vi "VIQA Find Legal Marking.vi"(8 "error in (no error)":errorcluster, 9 "Return Decor Refnum? (F)":bool, 10 "Ignore? (F)":bool, 11 "VI Refnum":refnum<vi>) -> (0 "error out":errorcluster, 1 "Found?":bool, 2 "Legal Marking":string, 3 "dup VI Refnum":refnum<vi>, 5 "Decor Refnum":refnum<vi>, 7 "Tag Name":string="BATC_SW_LEGALMARKING")   [LabVIEW 2018, in "VI Quality.lvlib"]
doc: "This VI finds the legal markings comment on the block diagram."
uses:
  VI Quality.lvlib
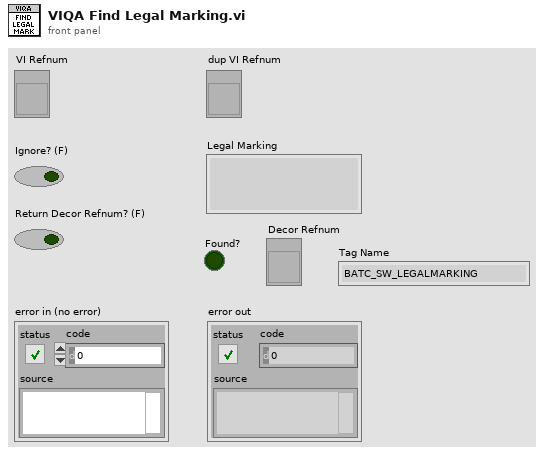
[diagram p1: front panel]
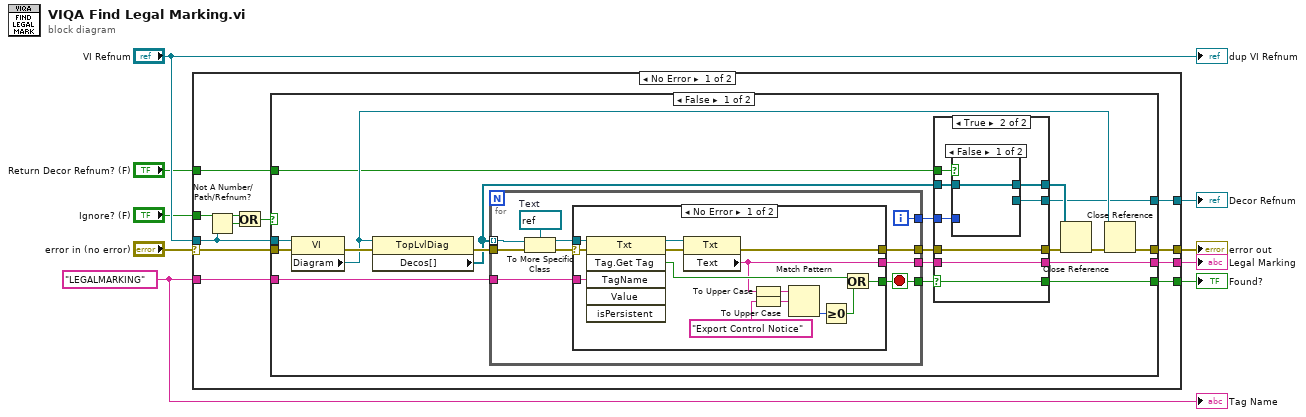
[diagram p0: block diagram]
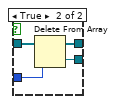
[diagram p3: hidden frame]
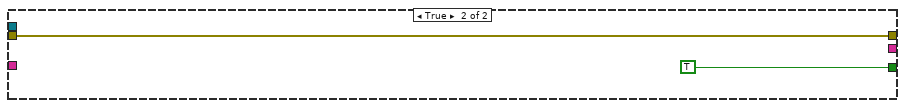
[diagram p5: hidden frame]
diagram:
  w9 = "LEGALMARKING" ("Tag Name")
  n1 = case shown="No Error" "error in (no error)" {
    selector: "error in (no error)" -> [w15 w82]
    tunnel: w9 -> [w20 _]
    tunnel: [w18 _] -> w8
    tunnel: [w17 _] -> w7
    tunnel: [w16 w82] -> w6
    tunnel: "VI Refnum" -> [w14 _]
    tunnel: "Ignore? (F)" -> [w12 _]
    tunnel: [w11 _] -> w2
    tunnel: "Return Decor Refnum? (F)" -> [w10 _]
    frame No Error {
      n2 = Not A Number/Path/Refnum?(number/path/refnum=w14) -> (NaN/Path/Refnum?=w19:bool)
      n3 = Or(x=w12, y=w19) -> (x .or. y?=w13:bool)
      n4 = case shown="False" w13 {
        tunnel: w20 -> [w39 _]
        tunnel: [w22 TRUE ("GetTag")] -> w18
        tunnel: w14 -> [w37 _]
        tunnel: [w24 _] -> w17
        tunnel: [w33 w80] -> w16
        tunnel: w15 -> [w32 w80]
        tunnel: [w26 _] -> w11
        tunnel: w10 -> [w21 _]
        frame False {
          n5 = property class="VI"(reference=w37, error in=w32) -> (error out=w35:errorcluster, "Diagram"=w34:refnum<vi>)  [unwired: 1 out]
          n6 = property class="TopLvlDiag"(reference=w34, error in=w35) -> (error out=w38:errorcluster, "Decos[]"=w31:refnum<vi>[])  [unwired: 1 out]
          n7 = for {
            tunnel: w31 -> [w62] mode=indexing
            tunnel: w39 -> [w65]
            tunnel: w38 -> [w64]
            tunnel: [w58] -> w23
            tunnel: [w59] -> w28
            tunnel: [w57] -> w25
            tunnel: [w56] -> w27
            i -> [w56]
            stop <- w58 stop-if-true
            w61 = refnum<vi> refnum  # Text
            n8 = To More Specific Class(target class=w61, reference=w62, error in=w64) -> (specific class reference=w60:refnum<vi>, error out=w63:errorcluster)
            n9 = case shown="No Error" w63 {
              selector: w63 -> [w78 _]
              tunnel: w65 -> [w79 _]
              tunnel: w60 -> [w77 _]
              tunnel: [w72 _] -> w59
              tunnel: [w67 _] -> w58
              tunnel: [w66 _] -> w57
              frame No Error {
                n10 = invoke class="Txt" method="Tag.Get Tag"(reference=w77, error in=w78, "TagName"=w79) -> (reference out=w71:refnum<vi>, error out=w73:errorcluster, "GetTag"=w68:bool)  [unwired: 3 in, 3 out]
                n11 = property class="Txt"(reference=w71, error in=w73) -> (error out=w72:errorcluster, "Text"=w66:string)  [unwired: 1 out]
                n12 = To Upper Case(1:w66) -> (0:w76:string)
                n13 = To Upper Case(1:"Export Control Notice" ("regular expression")) -> (0:w75:string)
                n14 = Match Pattern(string=w76, regular expression=w75) -> (offset past match=w70:i32)  [unwired: 1 in, 3 out]
                n15 = Greater Or Equal To 0?(x=w70) -> (x >= 0?=w69:bool)
                n16 = Or(x=w68, y=w69) -> (x .or. y?=w67:bool)
              }
              frame Error {
              }
            }
          }
          n17 = case shown="True" w23 {
            selector: w23 -> [w40 w44]
            tunnel: w31 -> [w42 w50]
            tunnel: [w42 w49] -> w30
            tunnel: [w41 w48] -> w29
            tunnel: w28 -> [w41 w48]
            tunnel: w27 -> [_ w47]
            tunnel: [_ w46] -> w26
            tunnel: w25 -> [_ w45]
            tunnel: [_ w45] -> w24
            tunnel: [w40 w44] -> w22
            tunnel: w21 -> [_ w43]
            frame False {
            }
            frame True {
              n18 = case shown="False" w43 {
                tunnel: w50 -> [w51 w55]
                tunnel: [w51 w54] -> w49
                tunnel: w47 -> [_ w53]
                tunnel: [_ w52] -> w46
                frame False {
                }
                frame True {
                  n19 = Delete From Array(array=w55, index=w53) -> (deleted portion=w52:refnum<vi>, array with subset deleted=w54:refnum<vi>[])  [unwired: 1 in]
                }
              }
            }
          }
          n20 = Close Reference(reference=w30, error in (no error)=w29) -> (error out=w36:errorcluster)
          n21 = Close Reference(reference=w34, error in (no error)=w36) -> (error out=w33:errorcluster)
        }
        frame True {
        }
      }
    }
    frame Error {
    }
  }
  "Found?" <- w8
  "Legal Marking" <- w7
  "error out" <- w6
  "Decor Refnum" <- w2
  "dup VI Refnum" <- "VI Refnum"
  "Tag Name" <- w9
